vi "RSZVB Initiate Source Power Calibration.vi"(7 "External Power Meter (0: No. 1)":i32(ring) items=["No. 1", "No. 2"], 8 "error in (no error)":errorcluster {"code" format="%.0x"}, 9 "Port Number (1)":i32=1, 10 "Channel (1)":i32=1, 11 "VISA session":refnum<visa-resource-name>) -> (0 "error out":errorcluster {"code" format="%.0x"}, 3 "dup VISA session":refnum<visa-resource-name>)   [LabVIEW 2011]
doc: "This VI initiates a source power calibration for the source port <pt> using an external power meter no. 1 or 2.\n\nNotes:\n\n(1) The VI cannot be used unless a power meter is connected via GPIB bus, USB or LAN interface and configured in the System - System Config - Configure External Power Meter.\n\n(2) For some measurements the default set timeout can be insufficient. To set higher timeout use VI RSZVB Set Time Out.vi.\n\nRemote-control command(s):\nSOURce<Ch>:POWer<Pt>:CORRection:COLLect[:ACQuire] ASENsor | BSENsor"
uses:
  _utility/RSZVB Global Data.vi
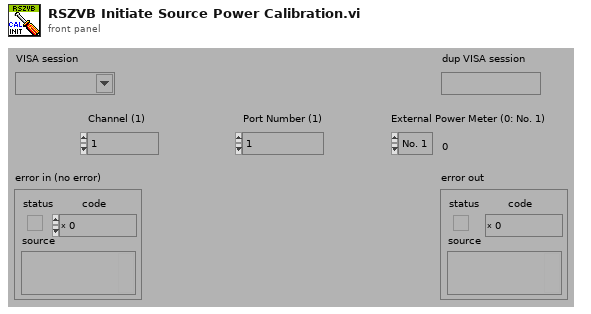
[diagram p1: front panel]
types:
  T1 = cluster{"Error Checking (T: On)":bool, "Installed Options":string[], "Data Valid?":bool, "Ports":i32, "Model":string[], "Option Checking (T: On)":bool}[]
  T2 = cluster{"Error Checking (T: On)":bool, "Installed Options":string[], "Data Valid?":bool, "Ports":i32, "Model":string[], "Option Checking (T: On)":bool}
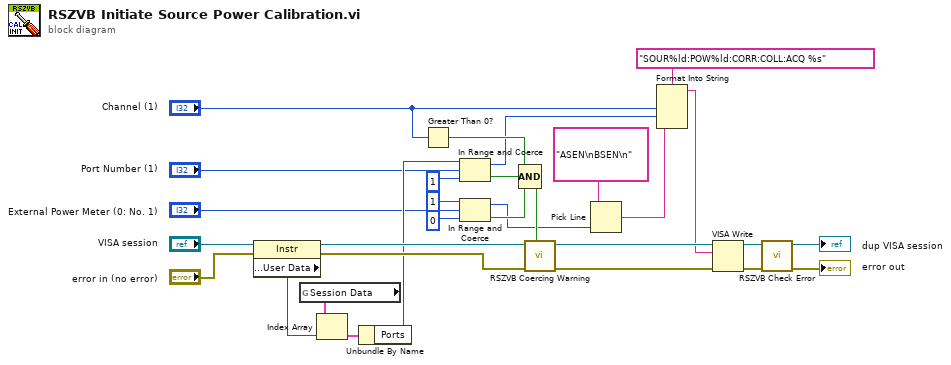
[diagram p0: block diagram]
diagram:
  n1 = property class="Instr"(reference="VISA session", error in="error in (no error)") -> (reference out=w16:refnum<visa-resource-name>, error out=w17:errorcluster, "General Settings:User Data"=w18:u32)
  n2 = global read "RSZVB Global Data.vi" "Session Data"() -> (w19:T1)
  n3 = Index Array(array=w19, index=w18) -> (element=w20:T2)
  n4 = Unbundle By Name(w20) -> ("Ports"=w13:i32)
  n5 = Greater Than 0?(x="Channel (1)") -> (x > 0?=w21:bool)
  n6 = In Range and Coerce(upper limit=w13, x="Port Number (1)", lower limit=1) -> (coerced(x)=w11:i32, In Range?=w24:bool)
  n7 = In Range and Coerce(upper limit=1 ("lower limit"), x="External Power Meter (0: No. 1)", lower limit=0) -> (coerced(x)=w9:i32, In Range?=w14:bool)
  n8 = Compound Arithmetic op=AND(w21, w24, w14) -> (w23:bool)
  n9 = call "RSZVB Coercing Warning.vi"("In Range?"=w23, "error in (no error)"=w17, "VISA session"=w16) -> ("error out"=w27:errorcluster, "dup VISA session"=w28:refnum<visa-resource-name>)  [unwired: 7 in]
  n10 = Pick Line(multi-line string="ASEN\nBSEN\n", line index=w9) -> (output string=w8:string)  [unwired: 1 in]
  n11 = Format Into String(format string="SOUR%ld:POW%ld:CORR:COLL:ACQ %s", "Channel (1)", w11, w8) -> (resulting string=w22:string)  [unwired: 2 in, 1 out]
  n12 = VISA Write(VISA resource name=w28, write buffer=w22, error in (no error)=w27) -> (VISA resource name out=w25:refnum<visa-resource-name>, error out=w26:errorcluster)  [unwired: 1 out]
  n13 = call "RSZVB Check Error.vi"("error in (no error)"=w26, "VISA session"=w25) -> ("error out"=→"error out":errorcluster, "dup VISA session"=→"dup VISA session":refnum<visa-resource-name>)  [unwired: 8 in]
